vi "Daemon.vi"(10 "error in (no error)":errorcluster, 11 "WAMP Client in":refnum<class "WAMP Client.lvclass">) -> (2 "error out":errorcluster, 3 "WAMP Client out":refnum<class "WAMP Client.lvclass">)   [LabVIEW 2020, in "WAMP Client.lvclass"]
uses:
  <userlib>/lvwamp/WAMP Client/WAMP Client.lvclass
  <userlib>/lvwamp/WAMP Client/TypeDef/SUBSCRIBE Request Data.ctl
  <userlib>/lvwamp/WAMP Client/TypeDef/SUBSCRIBE Result.ctl
  <userlib>/lvwamp/WAMP Client/TypeDef/EVENT Payload.ctl
  <userlib>/lvwamp/WAMP Client/TypeDef/Subscriptions Map.ctl
  <userlib>/lvwamp/WAMP Client/TypeDef/Subscription Details.ctl
  <userlib>/lvwamp/WAMP Client/TypeDef/Unsubscribe Requests Map.ctl
  <userlib>/lvwamp/WAMP Client/TypeDef/UNSUBSCRIBE Request Data.ctl
  <userlib>/lvwamp/WAMP Client/TypeDef/UNSUBSCRIBE Result.ctl
  <userlib>/lvwamp/WAMP Client/WAMP Client.lvclass/WAMP Client.ctl
  <userlib>/lvwamp/WAMP Client/TypeDef/Internal Message.ctl
  <userlib>/lvwamp/WAMP Client/TypeDef/Internal Message Type.ctl
  <userlib>/lvwamp/WAMP Client/TypeDef/WAMP Received Message.ctl
  <userlib>/lvwamp/WAMP Message Codes.ctl
  <userlib>/lvwamp/WAMP Client/TypeDef/PUBLISH Request Data.ctl
  <userlib>/lvwamp/WAMP Client/TypeDef/PUBLISH Result.ctl
  <vilib>/JDP Science/JSONtext/Get Array Elements.vi
  <userlib>/lvwamp/Comm Handlers/ICommHandler/ICommHandler.lvclass
panel:
  out "Stop Daemon?":bool
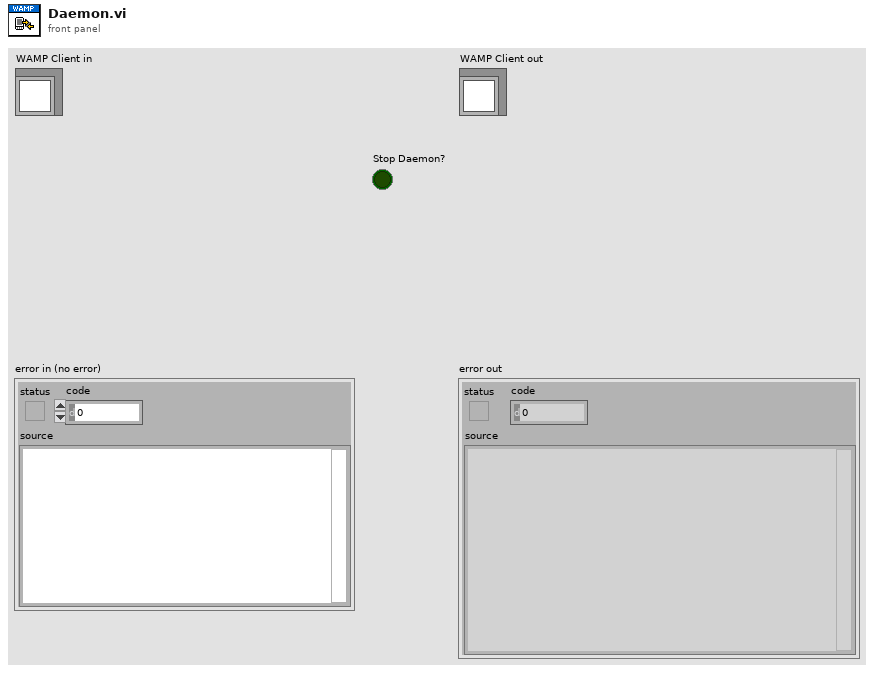
[diagram p1: front panel]
types:
  T1 = typedef "WAMP Client.lvclass/SUBSCRIBE Request Data.ctl" = cluster{"Topic":string, "Subscribe Response Received Event":refnum<user-event>}
  T2 = typedef "WAMP Client.lvclass/WAMP Received Message.ctl" = cluster{"Message JSON":string[], "Message Codes":T3}
  T3 = typedef "WAMP Client.lvclass/WAMP Message Codes.ctl" = u16
  T4 = typedef "WAMP Client.lvclass/UNSUBSCRIBE Request Data.ctl" = cluster{"Topic":string, "Unsubscribe Result Received Event":refnum<user-event>}
  T5 = typedef "WAMP Client.lvclass/PUBLISH Request Data.ctl" = cluster{"Topic URI":string, "Arguments":variant[], "ArgumentsKw":string, "Publish Result Event":refnum<user-event>}
  T6 = typedef "WAMP Client.lvclass/Internal Message Type.ctl" = enum16{"Subscribe", "Handle Subscribed", "Handle Event", "Unsubscribe", "Handle Unsubscribed", "Publish"}
  T7 = typedef "WAMP Client.lvclass/Internal Message.ctl" = cluster{"Internal Message Type":T6, "Variant":variant}
  T8 = typedef "WAMP Client.lvclass/Unsubscribe Requests Map.ctl" = map{u32, T4}
  T9 = typedef "WAMP Client.lvclass/Subscriptions Map.ctl" = map{u32, T10}
  T10 = typedef "WAMP Client.lvclass/Subscription Details.ctl" = cluster{"Subscription ID":u32, "Topic":string, "Publication Received Event":refnum<user-event>}
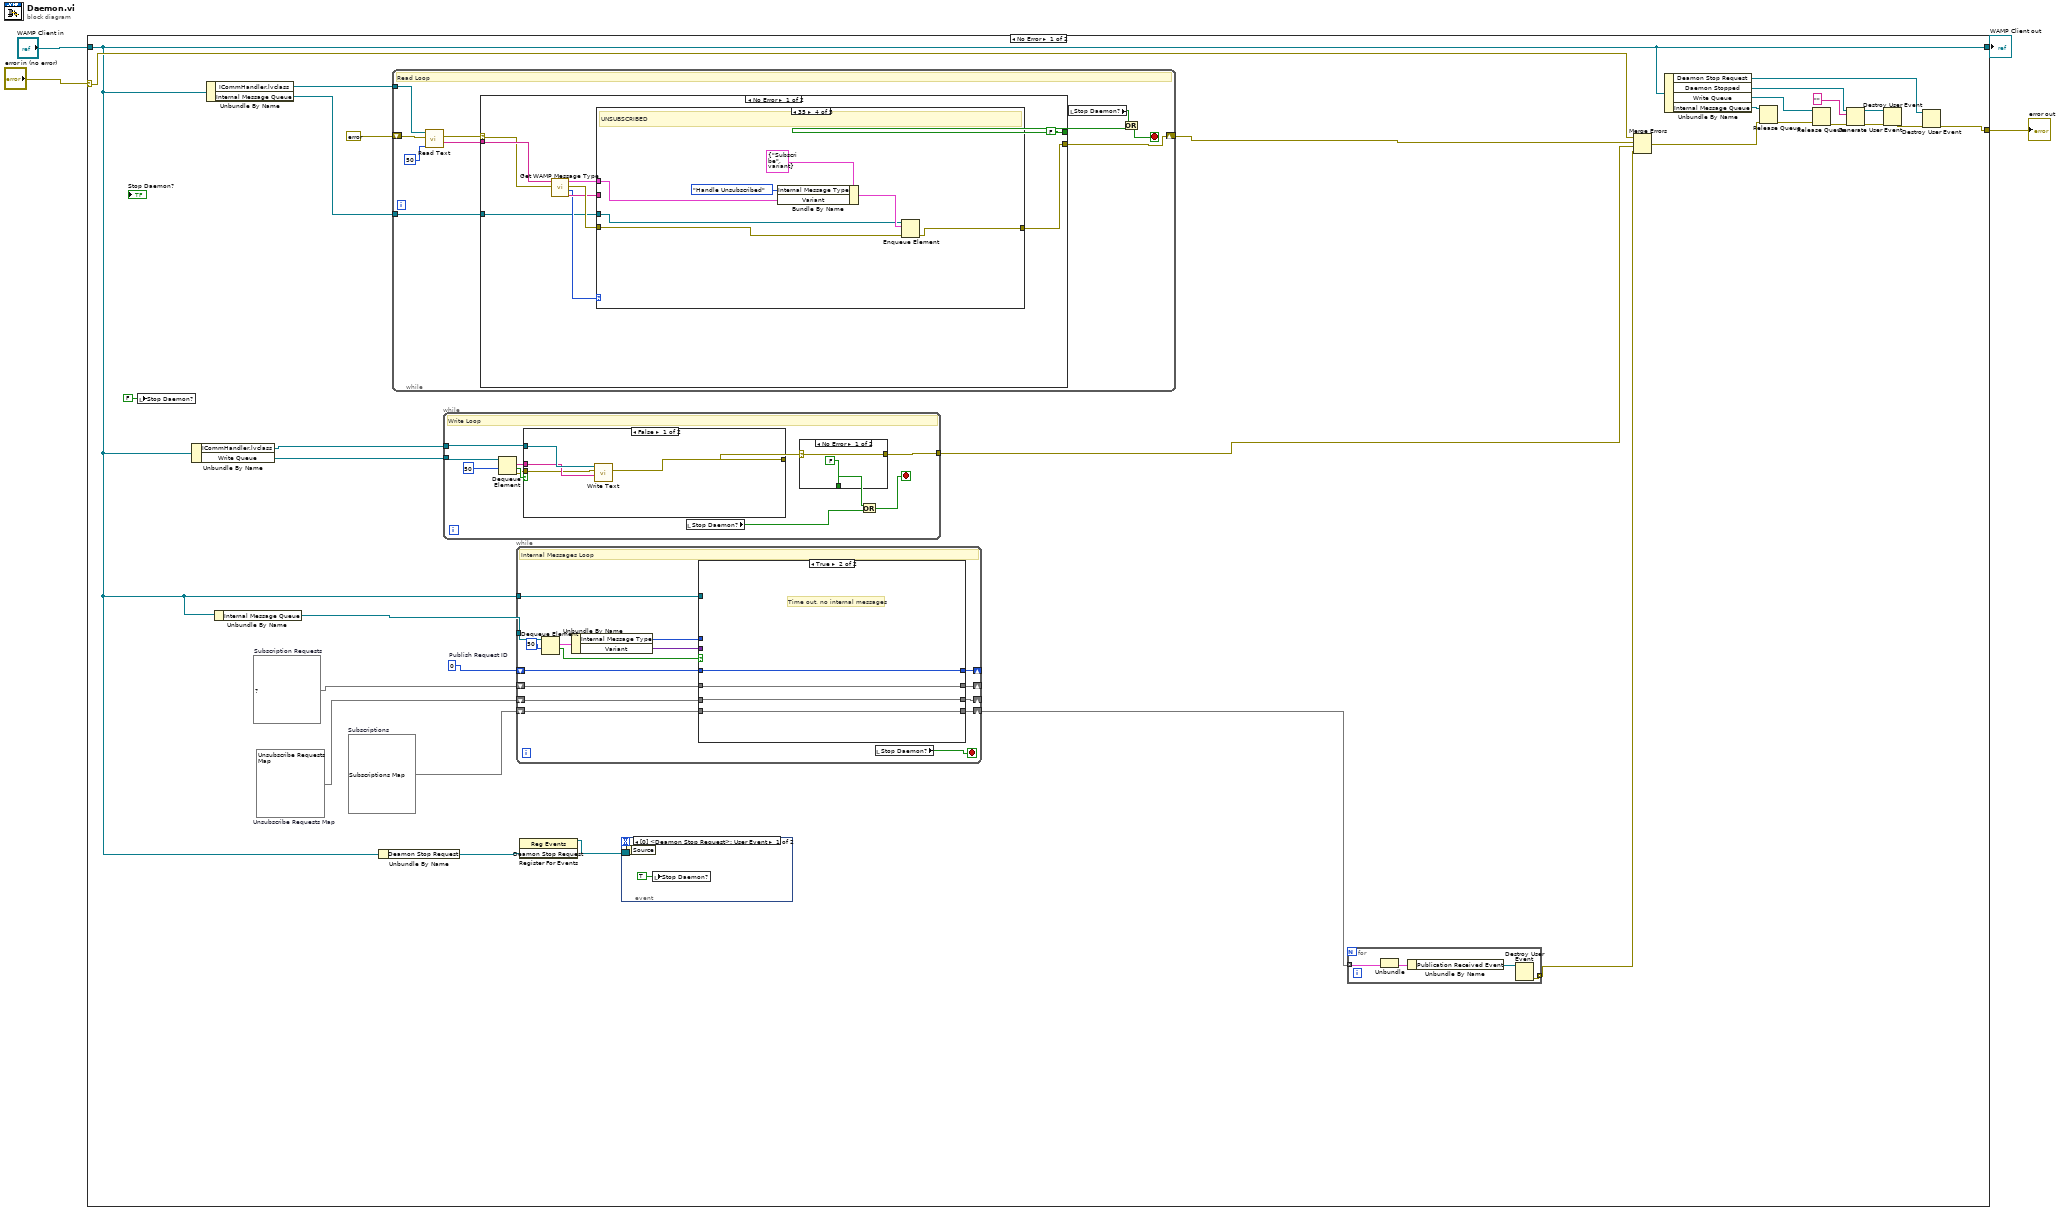
[diagram p0: block diagram]
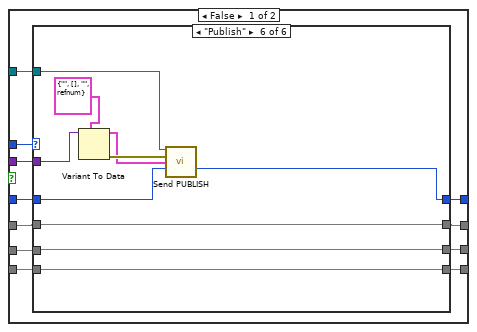
[diagram p2: hidden frame]
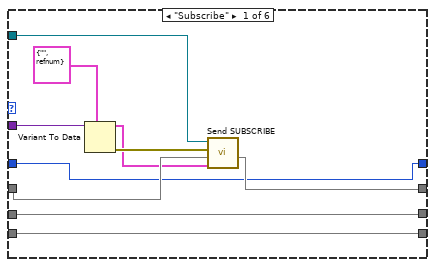
[diagram p3: hidden frame]
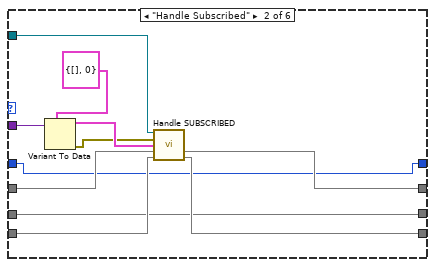
[diagram p4: hidden frame]
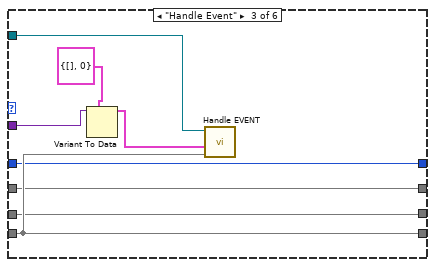
[diagram p5: hidden frame]
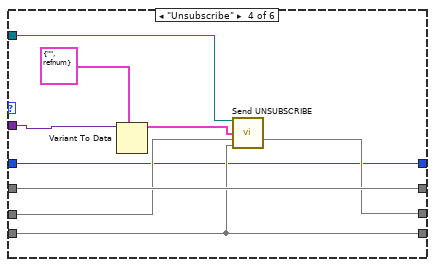
[diagram p6: hidden frame]
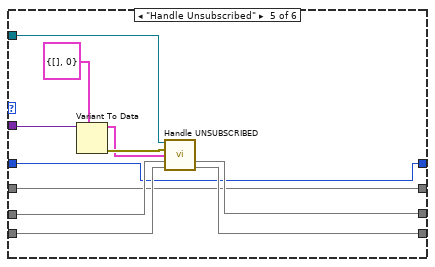
[diagram p7: hidden frame]
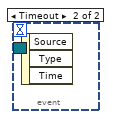
[diagram p8: hidden frame]
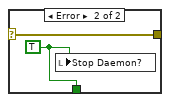
[diagram p9: hidden frame]
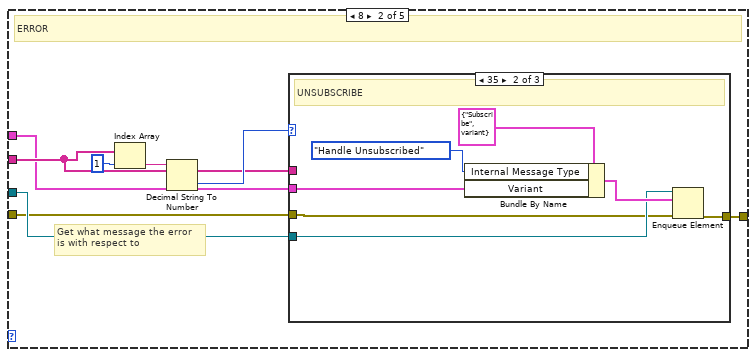
[diagram p12: hidden frame]
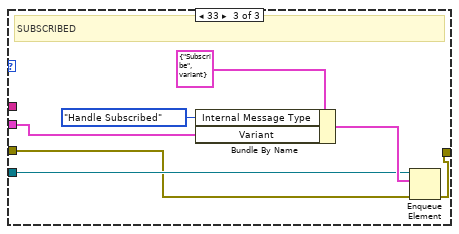
[diagram p14: hidden frame]
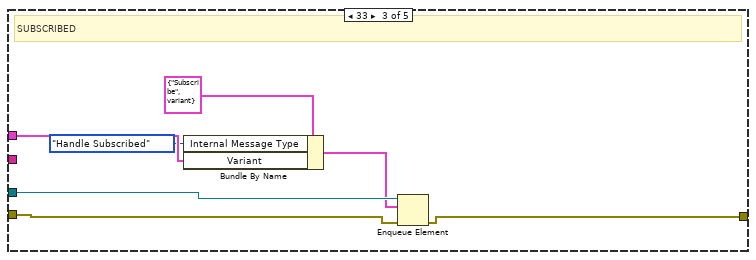
[diagram p15: hidden frame]
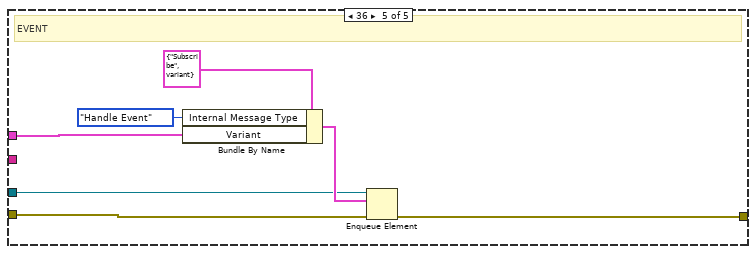
[diagram p16: hidden frame]
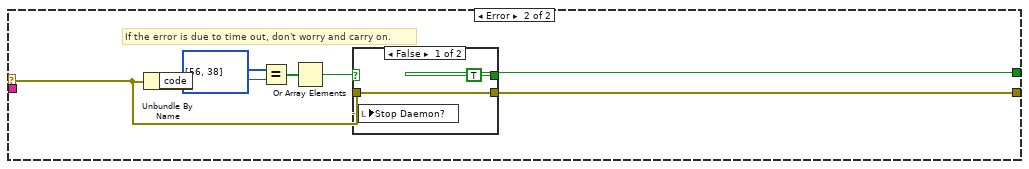
[diagram p17: hidden frame]
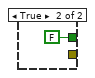
[diagram p18: hidden frame]
diagram:
  n1 = case shown="No Error" "error in (no error)" {
    selector: "error in (no error)" -> [w19 w226]
    tunnel: [w12 w226] -> w3
    tunnel: [w17 w225] -> w1
    tunnel: "WAMP Client in" -> [w17 w225]
    frame No Error {
      w5 = u32 0  # Publish Request ID
      w6 = T8 {}  # Unsubscribe Requests Map
      w29 = T9 {}  # Subscriptions
      w30 = map{u32, T1} {}  # Subscription Requests
      n2 = local write "Stop Daemon?"(FALSE ("Stop Daemon?")) -> ()
      n3 = Unbundle By Name(w17) -> ("ICommHandler.lvclass"=w23:refnum<class "ICommHandler.lvclass">, "Write Queue"=w24:refnum<queue>)
      n4 = Unbundle By Name(w17) -> ("ICommHandler.lvclass"=w31:refnum<class "ICommHandler.lvclass">, "Internal Message Queue"=w16:refnum<queue>)
      n5 = Unbundle By Name(w17) -> ("Internal Message Queue"=w22:refnum<queue>)
      n6 = Unbundle By Name(w17) -> ("Deamon Stop Request"=w18:refnum<user-event>)
      n7 = while {
        tunnel: w31 -> [w159]
        shift-right: [w151] -> w20
        shift-left: errorcluster {"status"=FALSE, "code"=0, "source"=""} ("error IO") -> [w158]
        tunnel: w16 -> [w150]
        stop <- w154 stop-if-true
        # "Read Loop"
        n8 = call-dynamic "Read Text.vi"("timeout ms (5000)"=50, "error in (no error)"=w158, "ICommHandler in"=w159) -> ("String"=w152:string, "error out"=w156:errorcluster)  [unwired: 4 in, 1 out]
        n9 = case shown="No Error" w156 {
          selector: w156 -> [w162 w220]
          tunnel: [w160 w219] -> w151
          tunnel: [FALSE w218] -> w155
          tunnel: w152 -> [w163 _]
          tunnel: w150 -> [w161 _]
          frame No Error {
            n10 = call <userlib>:"Get WAMP Message Type.vi"("error in (no error)"=w162, "JSON"=w163) -> ("<JSON>"=w165:string[], "Message Codes"=w164:T3, "error out"=w166:errorcluster, "WAMP Message"=w167:T2)  [unwired: 6 in]
            n11 = case shown="35" w164 {
              tunnel: w165 -> [_ w174 _ _ _]
              tunnel: w166 -> [w169 w171 w194 w202 w209]
              tunnel: w161 -> [_ w172 w199 w201 w210]
              tunnel: w167 -> [_ w173 w196 w204 w211]
              tunnel: [w169 w170 w195 w203 w208] -> w160
              frame 0, Default {
              }
              frame 8 {
                # "Get what message the error \nis with respect to"
                # "ERROR"
                n12 = Index Array(array=w174, index=1) -> (element=w176:string)
                n13 = Decimal String To Number(string=w176) -> (number=w175:i32)  [unwired: 2 in, 1 out]
                n14 = case shown="35" w175 {
                  tunnel: w174 -> [_ _ _]
                  tunnel: w173 -> [_ w182 w190]
                  tunnel: w172 -> [_ w181 w189]
                  tunnel: w171 -> [w178 w180 w188]
                  tunnel: [w178 w179 w187] -> w170
                  frame 0, Default {
                  }
                  frame 35 {
                    # "UNSUBSCRIBE"
                    n15 = Bundle By Name(cluster=T7 {"Internal Message Type"=enum."Subscribe", "Variant"=variant} ("Cluster"), "Internal Message Type"=Internal_Message_Type."Handle Unsubscribed", "Variant"=w182) -> (w184:T7)
                    n16 = Enqueue Element(queue=w181, element=w184, error in (no error)=w180) -> (error out=w179:errorcluster)  [unwired: 1 in, 2 out]
                  }
                  frame 33 {
                    # "SUBSCRIBED"
                    n17 = Bundle By Name(cluster=T7 {"Internal Message Type"=enum."Subscribe", "Variant"=variant} ("Cluster"), "Internal Message Type"=Internal_Message_Type."Handle Subscribed", "Variant"=w190) -> (w191:T7)
                    n18 = Enqueue Element(queue=w189, element=w191, error in (no error)=w188) -> (error out=w187:errorcluster)  [unwired: 1 in, 2 out]
                  }
                }
              }
              frame 33 {
                # "SUBSCRIBED"
                n19 = Bundle By Name(cluster=T7 {"Internal Message Type"=enum."Subscribe", "Variant"=variant} ("Cluster"), "Internal Message Type"=Internal_Message_Type."Handle Subscribed", "Variant"=w196) -> (w197:T7)
                n20 = Enqueue Element(queue=w199, element=w197, error in (no error)=w194) -> (error out=w195:errorcluster)  [unwired: 1 in, 2 out]
              }
              frame 35 {
                # "UNSUBSCRIBED"
                n21 = Bundle By Name(cluster=T7 {"Internal Message Type"=enum."Subscribe", "Variant"=variant} ("Cluster"), "Internal Message Type"=Internal_Message_Type."Handle Unsubscribed", "Variant"=w204) -> (w205:T7)
                n22 = Enqueue Element(queue=w201, element=w205, error in (no error)=w202) -> (error out=w203:errorcluster)  [unwired: 1 in, 2 out]
              }
              frame 36 {
                # "EVENT"
                n23 = Bundle By Name(cluster=T7 {"Internal Message Type"=enum."Subscribe", "Variant"=variant} ("Cluster"), "Internal Message Type"=Internal_Message_Type."Handle Event", "Variant"=w211) -> (w212:T7)
                n24 = Enqueue Element(queue=w210, element=w212, error in (no error)=w209) -> (error out=w208:errorcluster)  [unwired: 1 in, 2 out]
              }
            }
          }
          frame Error {
            # "If the error is due to time out, don't worry and carry on."
            n25 = Unbundle By Name(w220) -> ("code"=w217:i32)
            n26 = Equal?(x=i32[] [56, 38] ("y"), y=w217) -> (x = y?=w215:bool[])
            n27 = Or Array Elements(Boolean array=w215) -> (logical OR=w214:bool)
            n28 = case shown="False" w214 {
              selector: w214 -> [w222 _]
              tunnel: w220 -> [w223 _]
              tunnel: [w223 _] -> w219
              tunnel: [TRUE FALSE] -> w218
              frame False {
                n29 = local write "Stop Daemon?"(w222) -> ()
              }
              frame True {
              }
            }
          }
        }
        n30 = local read "Stop Daemon?"() -> (w153:bool)
        n31 = Or(x=w153, y=w155) -> (x .or. y?=w154:bool)
      }
      n32 = while {
        tunnel: w24 -> [w141]
        tunnel: w23 -> [w140]
        tunnel: [w135] -> w35
        stop <- w132 stop-if-true
        # "Write Loop"
        n33 = Dequeue Element(queue=w141, timeout in ms (-1)=50) -> (element=w139:string, timed out?=w138:bool, error out=w137:errorcluster)  [unwired: 1 in, 1 out]
        n34 = case shown="False" w138 {
          tunnel: w140 -> [w149 _]
          tunnel: w139 -> [w148 _]
          tunnel: w137 -> [w147 _]
          tunnel: [w146 _] -> w136
          frame False {
            n35 = call-dynamic "Write Text.vi"("String"=w148, "error in (no error)"=w147, "ICommHandler in"=w149) -> ("error out"=w146:errorcluster)  [unwired: 7 in, 1 out]
          }
          frame True {
            # "Queue is empty, do nothing"
          }
        }
        n36 = local read "Stop Daemon?"() -> (w131:bool)
        n37 = case shown="No Error" w136 {
          selector: w136 -> [w142 w145]
          tunnel: [FALSE w144] -> w133
          tunnel: [w142 w145] -> w135
          frame No Error {
          }
          frame Error {
            w144 = TRUE ("Stop Daemon?")
            n38 = local write "Stop Daemon?"(w144) -> ()
          }
        }
        n39 = Or(x=w133, y=w131) -> (x .or. y?=w132:bool)
      }
      n40 = while {
        tunnel: w22 -> [w54]
        tunnel: w17 -> [w50]
        shift-right: [w48] -> _
        shift-left: w30 -> [w49]
        shift-right: [w46] -> w28
        shift-left: w29 -> [w47]
        shift-right: [w43] -> _
        shift-left: w6 -> [w44]
        shift-right: [w40] -> _
        shift-left: w5 -> [w41]
        stop <- w45 stop-if-true
        # "Internal Messages Loop"
        n41 = Dequeue Element(queue=w54, timeout in ms (-1)=50) -> (element=w53:T7, timed out?=w42:bool)  [unwired: 1 in, 2 out]
        n42 = Unbundle By Name(w53) -> ("Internal Message Type"=w52:T6, "Variant"=w51:variant)
        n43 = case shown="True" w42 {
          tunnel: w52 -> [w66 _]
          tunnel: w51 -> [w65 _]
          tunnel: w50 -> [w64 _]
          tunnel: w49 -> [w63 w129]
          tunnel: [w62 w129] -> w48
          tunnel: w47 -> [w61 w127]
          tunnel: [w60 w127] -> w46
          tunnel: w44 -> [w59 w128]
          tunnel: [w58 w128] -> w43
          tunnel: w41 -> [w57 w126]
          tunnel: [w56 w126] -> w40
          frame False {
            n44 = case shown="\"Publish\"" w66 {
              tunnel: w65 -> [w76 w86 w92 w104 w115 w118]
              tunnel: w64 -> [w74 w87 w95 w102 w113 w119]
              tunnel: w63 -> [w72 w82 w93 w103 w106 w125]
              tunnel: [w71 w80 w93 w103 w106 w125] -> w62
              tunnel: w61 -> [w69 w81 w94 w97 w108 w123]
              tunnel: [w69 w79 w94 w97 w107 w123] -> w60
              tunnel: w59 -> [w68 w78 w89 w99 w110 w124]
              tunnel: [w68 w78 w89 w98 w109 w124] -> w58
              tunnel: w57 -> [w67 w77 w88 w96 w105 w122]
              tunnel: [w67 w77 w88 w96 w105 w121] -> w56
              frame "Subscribe" {
                n45 = Variant To Data(type=T1 {"Topic"="", "Subscribe Response Received Event"=refnum} ("Cluster"), Variant=w76) -> (data=w70:T1, error out=w73:errorcluster)  [unwired: 1 in]
                n46 = call-dynamic "Send SUBSCRIBE.vi"("Subscription Request"=w70, "Subscription Requests Map"=w72, "error in (no error)"=w73, "WAMP Client in"=w74) -> ("Subscription Requests List 2"=w71:map{u32, T1})  [unwired: 5 in, 2 out]
              }
              frame "Handle Subscribed" {
                n47 = Variant To Data(type=T2 {"Message JSON"=[], "Message Codes"=0} ("Cluster"), Variant=w86) -> (data=w84:T2, error out=w83:errorcluster)  [unwired: 1 in]
                n48 = call-dynamic "Handle SUBSCRIBED.vi"("reference"=w87, "error in (no error)"=w83, "WAMP Message"=w84, "Subscription Requests In"=w82, "Subscriptions In"=w81) -> ("Subscription Requests Out"=w80:map{u32, T1}, "Subscriptions Map Out"=w79:map{u32, T10})  [unwired: 7 in, 2 out]
              }
              frame "Handle Event" {
                n49 = Variant To Data(type=T2 {"Message JSON"=[], "Message Codes"=0} ("Cluster"), Variant=w92) -> (data=w91:T2)  [unwired: 1 in, 1 out]
                n50 = call-dynamic "Handle EVENT.vi"("Subscriptions"=w94, "Cluster"=w91, "reference"=w95) -> ()  [unwired: 7 in, 2 out]
              }
              frame "Unsubscribe" {
                n51 = Variant To Data(type=T4 {"Topic"="", "Unsubscribe Result Received Event"=refnum} ("Cluster"), Variant=w104) -> (data=w101:T4)  [unwired: 1 in, 1 out]
                n52 = call-dynamic "Send UNSUBSCRIBE.vi"("WAMP Client in"=w102, "Unsubscribe Request Data"=w101, "Unsubscribe Requests Map (in)"=w99, "Subscriptions"=w97) -> ("Unsubscribe Requests Map (out)"=w98:T8)  [unwired: 9 in, 2 out]
              }
              frame "Handle Unsubscribed" {
                n53 = Variant To Data(type=T2 {"Message JSON"=[], "Message Codes"=0} ("Cluster"), Variant=w115) -> (data=w111:T2, error out=w112:errorcluster)  [unwired: 1 in]
                n54 = call-dynamic "Handle UNSUBSCRIBED.vi"("reference"=w113, "error in (no error)"=w112, "WAMP Message"=w111, "Unsubscribe Reqeusts (in)"=w110, "Subscriptions In"=w108) -> ("Unsubscribe Reqeusts (out)"=w109:T8, "Subscriptions Map Out"=w107:map{u32, T10})  [unwired: 7 in, 2 out]
              }
              frame "Publish" {
                n55 = Variant To Data(type=T5 {"Topic URI"="", "Arguments"=[], "ArgumentsKw"="", "Publish Result Event"=refnum} ("Cluster"), Variant=w118) -> (data=w116:T5, error out=w120:errorcluster)  [unwired: 1 in]
                n56 = call-dynamic "Send PUBLISH.vi"("WAMP Client in"=w119, "error in (no error)"=w120, "Publish Request Data"=w116, "Publish Request ID"=w122) -> ("Publish Request ID (out)"=w121:u32)  [unwired: 9 in, 2 out]
              }
            }
          }
          frame True {
            # "Time out, no internal messages"
          }
        }
        n57 = local read "Stop Daemon?"() -> (w45:bool)
      }
      n58 = register-events(w18) -> (reference out=w33:refnum<event-registration>)  [unwired: 2 in, 1 out]
      n59 = event shown="[0] <Deamon Stop Request>: User Event" {
        selector: w33 -> [_ _]
        dyn-events: _ -> [_ _]
        timeout: _ -> [_ _]
        event User Event {
          n60 = event-data() -> ()  [unwired: 1 in, 1 out]
          n61 = local write "Stop Daemon?"(TRUE ("Stop Daemon?")) -> ()
        }
        event Timeout {
          n62 = event-data() -> ()  [unwired: 1 in, 3 out]
        }
      }
      n63 = for {
        tunnel: w28 -> [w39] mode=indexing
        tunnel: [w36] -> w25 mode=indexing
        n64 = Unbundle(w39) -> (w38:T10)  [unwired: 1 out]
        n65 = Unbundle By Name(w38) -> ("Publication Received Event"=w37:refnum<user-event>)
        n66 = Destroy User Event(user event=w37) -> (error out=w36:errorcluster)  [unwired: 1 in]
      }
      n67 = Merge Errors(w19, w20, w35, w25) -> (w7:errorcluster)
      n68 = Unbundle By Name(w17) -> ("Deamon Stop Request"=w15:refnum<user-event>, "Daemon Stopped"=w14:refnum<user-event>, "Write Queue"=w11:refnum<queue>, "Internal Message Queue"=w10:refnum<queue>)
      n69 = Release Queue(queue=w10, error in (no error)=w7) -> (error out=w9:errorcluster)  [unwired: 1 in, 2 out]
      n70 = Release Queue(queue=w11, error in (no error)=w9) -> (error out=w8:errorcluster)  [unwired: 1 in, 2 out]
      n71 = Generate User Event(user event=w14, event data cluster="" ("event data"), error in=w8) -> (user event out=w27:refnum<user-event>, error out=w26:errorcluster)  [unwired: 1 in]
      n72 = Destroy User Event(user event=w27, error in=w26) -> (error out=w13:errorcluster)
      n73 = Destroy User Event(user event=w15, error in=w13) -> (error out=w12:errorcluster)
    }
    frame Error {
    }
  }
  "error out" <- w3
  "WAMP Client out" <- w1
